vi "WindowHandleCaptureSubVI.vi"(8 "error in (no error)":errorcluster, 10 "Path":string, 11 "Handle":i32) -> (0 "error out":errorcluster)   [LabVIEW 2013]
uses:
  C:/Perforce/LabVIEWTestSystems/LV GUI ToolKit/LV GUI 2013/LabVIEW GUI Automation Toolkit/Utility/User32Wrapper/User32Wrapper/bin/Release/User32Wrapper.dll
panel:
  out "return type":u32
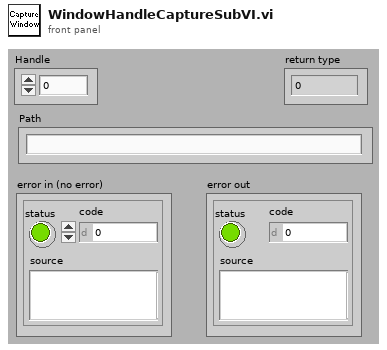
[diagram p1: front panel]
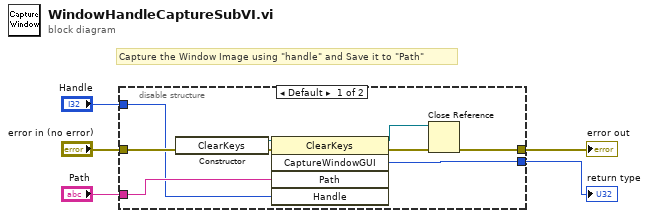
[diagram p0: block diagram]
diagram:
  # "Capture the Window Image using \"handle\" and Save it to \"Path\""
  n1 = disable-structure shown="Default" {
    disable-tunnel: "Path" -> [w12 _]
    disable-tunnel: "error in (no error)" -> [w11 w15]
    disable-tunnel: [w10 _] -> w2
    disable-tunnel: [w6 w15] -> w3
    disable-tunnel: "Handle" -> [w9 _]
    frame condition #0 (active) {
      n2 = constructor class="ClearKeys"(error in=w11) -> (reference out=w14:refnum<k24>, error out=w13:errorcluster)  [unwired: 2 in, 1 out]
      n3 = invoke class="ClearKeys" method="CaptureWindowGUI"(reference=w14, error in=w13, "Path"=w12, "Handle"=w9) -> (reference out=w8:refnum<k24>, error out=w7:errorcluster, "CaptureWindowGUI"=w10:i32)  [unwired: 1 in, 2 out]
      n4 = Close Reference(reference=w8, error in (no error)=w7) -> (error out=w6:errorcluster)
    }
    frame condition #1 {
      # "#ToDo - InFuture"
    }
  }
  "error out" <- w3
  "return type" <- w2
